vi "Constructor.vi"(6 "Message Queue":refnum<class "Delacor_lib_QMH_Message Queue.lvclass">, 8 "error in (no error)":errorcluster, 9 "Module ID":i32=-1, 10 "Connection ID":refnum<k5>, 11 "GenNet Variant Protocol in":refnum<class "GenNet Variant Protocol.lvclass">) -> (0 "error out":errorcluster, 3 "GenNet Variant Protocol out":refnum<class "GenNet Variant Protocol.lvclass">)   [LabVIEW 2020, in "hse-gennet.lvlib" / "GenNet Variant Protocol.lvclass"]
doc: "____\nHAMPEL SOFTWARE ENGINEERING v3.8.0 (2023-12-18 14:41)"
uses:
  GenNet Variant Protocol.lvclass
  <vilib>/Delacor/Delacor QMH/Libraries/Message Queue_class/Delacor_lib_QMH_Message Queue.lvclass
  GenNet Protocol.lvclass
  GenNet Variant Protocol.lvclass/GenNet Variant Protocol.ctl
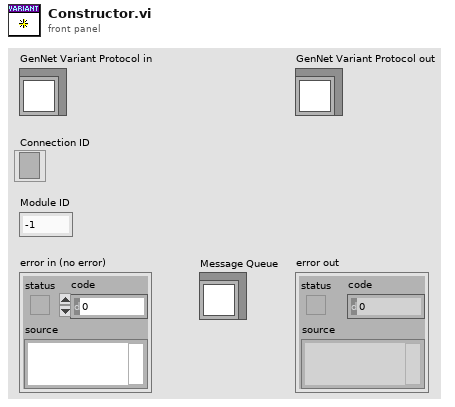
[diagram p1: front panel]
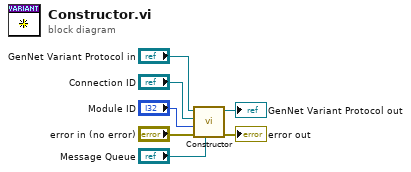
[diagram p0: block diagram]
diagram:
  n1 = call-parent "Constructor.vi"("Message Queue"="Message Queue", "error in (no error)"="error in (no error)", "Module ID"="Module ID", "Connection ID"="Connection ID", "GenNet Protocol in"="GenNet Variant Protocol in") -> ("error out"=→"error out":errorcluster, "GenNet Protocol out"=→"GenNet Variant Protocol out":refnum<class "GenNet Variant Protocol.lvclass">)  [unwired: 5 in]
